vi "Init Target Instrument.vi"(8 "error in (no error)":errorcluster, 9 "<JSON CFG>":string, 10 "Physical Instr CFGs":string[](array[string]), 11 "IHost Measure and Stimulus Subsystems in":refnum<class "ICRIO MSS Test Actor.lvclass">) -> (0 "error out":errorcluster, 3 "IHost Measure and Stimulus Subsystems out":refnum<class "ICRIO MSS Test Actor.lvclass">)   [LabVIEW 2023, in "ICRIO MSS Test Actor.lvlib" / "ICRIO MSS Test Actor.lvclass"]
uses:
  ICRIO MSS Test Actor.lvclass
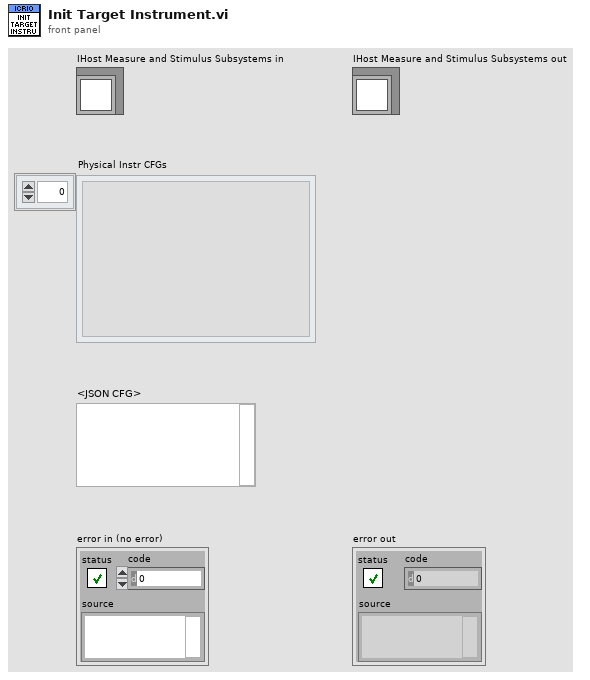
[diagram p1: front panel]
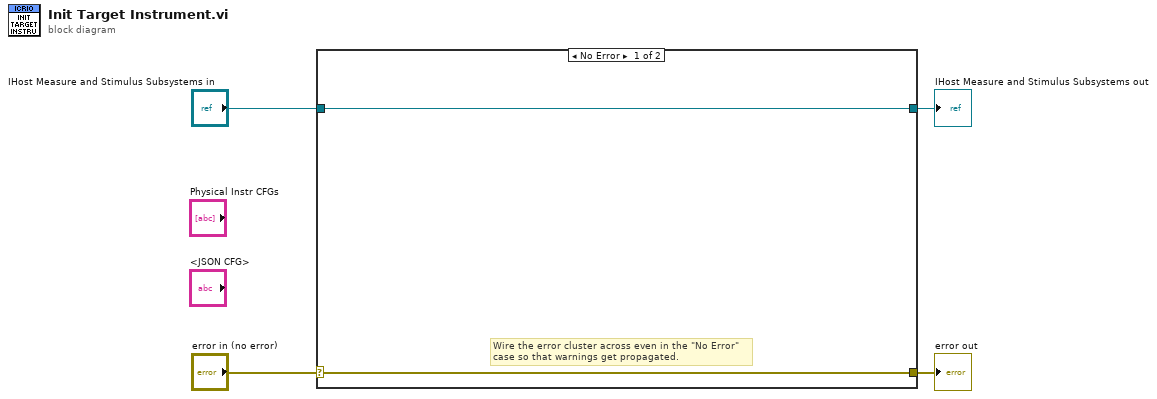
[diagram p0: block diagram]
diagram:
  n1 = case shown="No Error" "error in (no error)" {
    selector: "error in (no error)" -> [w5 w8]
    tunnel: [w5 w8] -> w3
    tunnel: [w6 w7] -> w1
    tunnel: "IHost Measure and Stimulus Subsystems in" -> [w6 w7]
    frame No Error {
      # "Wire the error cluster across even in the \"No Error\"\ncase so that warnings get propagated."
    }
    frame Error {
    }
  }
  "error out" <- w3
  "IHost Measure and Stimulus Subsystems out" <- w1
